vi "Gamepad PC.vi"() -> ()   [LabVIEW 2020]
uses:
  <vilib>/Utility/inputDevices.llb/closeJoystick.vi
panel:
  in  "stop":bool
  out "X Left":dbl(slide) scale=0.0..100.0
  out "nY Left":dbl(slide)
  out "Y Left":dbl(slide) scale=0.0..100.0
  out "nX Left":dbl(slide)
  out "X Right 2":dbl(slide) scale=0.0..100.0
  out "nY Right":dbl(slide)
  out "Z Left":dbl(slide)
  out "Z Right":dbl(slide) scale=0.0..100.0
  out "Y Right":dbl(slide) scale=0.0..100.0
  out "nX Right":dbl(slide)
  out "LB":bool
  out "RB":bool
  out "Back":bool
  out "Start":bool
  out "0":bool
  out "315":bool
  out "270":bool
  out "225":bool
  out "180":bool
  out "135":bool
  out "90":bool
  out "45":bool
  out "B":bool caption="Boolean"
  out "Y":bool caption="Boolean"
  out "A":bool caption="Boolean"
  out "X":bool caption="Boolean"
  out "R Stick":bool caption="Boolean"
  out "L Stick":bool caption="Boolean"
  out "error out":errorcluster
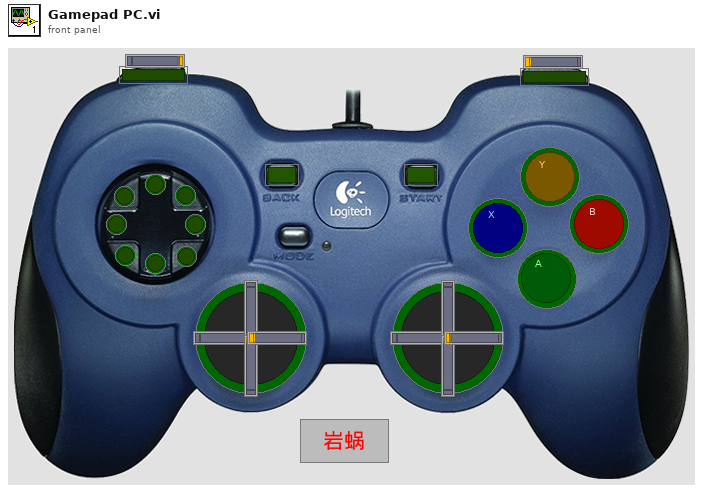
[diagram p1: front panel]
types:
  T1 = cluster{"axes total":u32, "buttons total":u32, "pov total":u32, "device name":string}[]
  T2 = typedef "Joystick controls.ctl" = cluster{"L Stick":bool, "R Stick":bool, "X":bool, "A":bool, "Y":bool, "B":bool, "45":bool, "90":bool, "135":bool, "180":bool, "225":bool, "270":bool, "315":bool, "0":bool, "Start":bool, "Back":bool, "RB":bool, "LB":bool, "X Right":i8, "Y Right":i8, "X Left":i8, "Y Left":i8, "Z Right":i8, "Pov":i16, "Z Left":i8, "Num":i16}
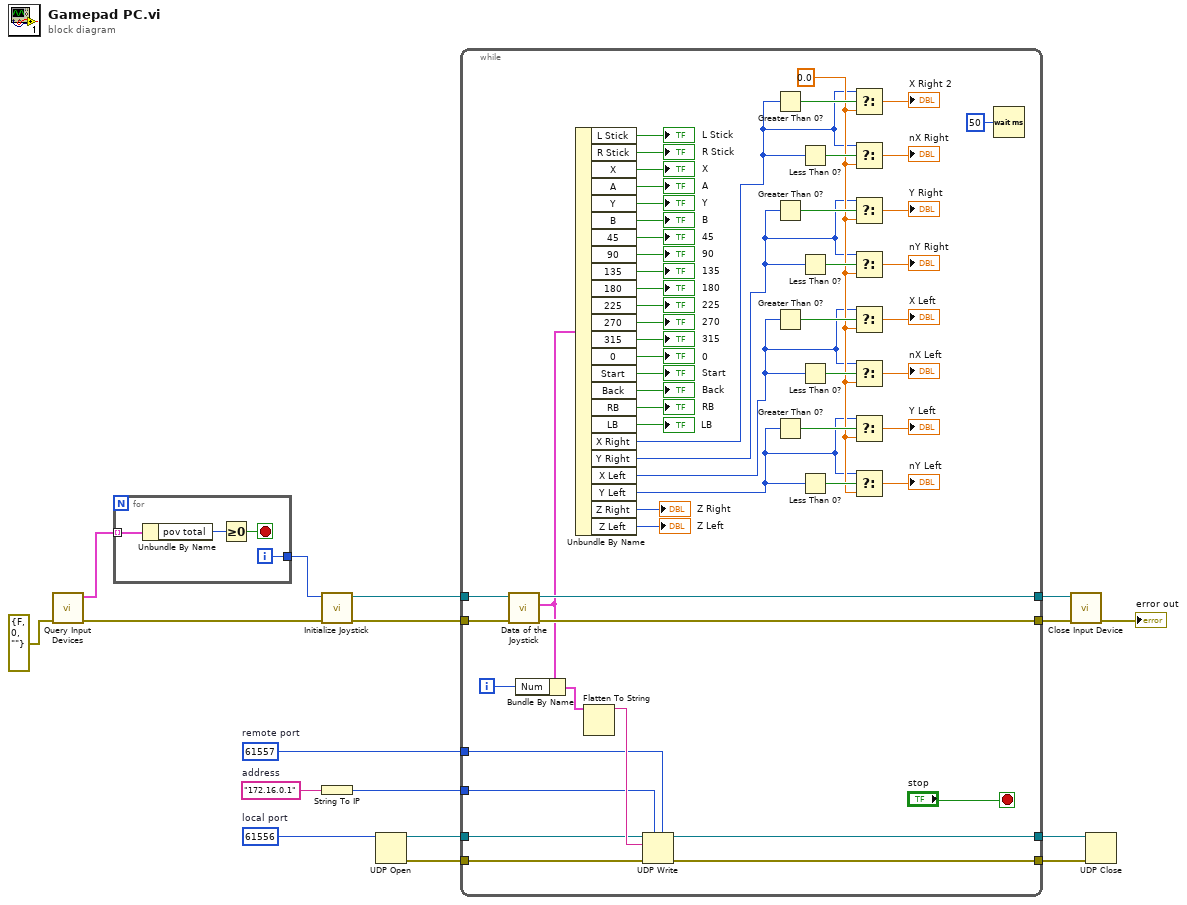
[diagram p0: block diagram]
diagram:
  w8 = "172.16.0.1"  # address
  w6 = u16 61557  # remote port
  w7 = u16 61556  # local port
  n1 = call <vilib>:"Query Input Devices.vi"("error in (no error)"=errorcluster {"status"=FALSE, "code"=0, "source"=""}) -> ("error out"=w9:errorcluster, "joystick info"=w11:T1)  [unwired: 7 in, 2 out]
  n2 = for {
    tunnel: w11 -> [w21] mode=indexing
    tunnel: [w18] -> w10
    i -> [w18]
    stop <- w20 stop-if-true
    n3 = Unbundle By Name(w21) -> ("pov total"=w19:u32)
    n4 = Greater Or Equal To 0?(x=w19) -> (x >= 0?=w20:bool)
  }
  n5 = call <vilib>:"Initialize Joystick.vi"("error in (no error)"=w9, "device index"=w10) -> ("error out"=w17:errorcluster, "device ID"=w14:refnum<k1>)  [unwired: 8 in]
  n6 = String To IP(1:w8) -> (0:w5:u32)
  n7 = UDP Open(11:w7) -> (port=w4:refnum<k16>, 0:w3:errorcluster)  [unwired: 4 in, 1 out]
  n8 = while {
    tunnel: w17 -> [w67]
    tunnel: [w66] -> w16
    tunnel: w14 -> [w68]
    tunnel: [w65] -> w13
    tunnel: w6 -> [w28]
    tunnel: w5 -> [w27]
    tunnel: w4 -> [w26]
    tunnel: w3 -> [w25]
    tunnel: [w23] -> w2
    tunnel: [w22] -> w1
    i -> [w30]
    stop <- "stop" stop-if-true
    w36 = 0.0 ("t")
    n9 = call "Data of the Joystick.vi"("error in (no error)"=w67, "device ID"=w68) -> ("error out"=w66:errorcluster, "Joystick"=w31:T2, "device ID out"=w65:refnum<k1>)  [unwired: 7 in]
    n10 = Bundle By Name(cluster=w31, "Num"=w30) -> (w24:T2)
    n11 = Unbundle By Name(w31) -> ("L Stick"=→"L Stick":bool, "R Stick"=→"R Stick":bool, "X"=→"X":bool, "A"=→"A":bool, "Y"=→"Y":bool, "B"=→"B":bool, "45"=→"45":bool, "90"=→"90":bool, "135"=→"135":bool, "180"=→"180":bool, "225"=→"225":bool, "270"=→"270":bool, "315"=→"315":bool, "0"=→"0":bool, "Start"=→"Start":bool, "Back"=→"Back":bool, "RB"=→"RB":bool, "LB"=→"LB":bool, "X Right"=w35:i8, "Y Right"=w34:i8, "X Left"=w33:i8, "Y Left"=w32:i8, "Z Right"=→"Z Right":i8, "Z Left"=→"Z Left":i8)
    n12 = Flatten To String(anything=w24) -> (data string=w29:string)  [unwired: 3 in, 2 out]
    n13 = UDP Write(address=w27, port or service name=w28, connection ID=w26, data in=w29, 8:w25) -> (error out=w23:errorcluster, 3:w22:refnum<k16>)  [unwired: 1 in]
    n14 = Greater Than 0?(x=w35) -> (x > 0?=w77:bool)
    n15 = Greater Than 0?(x=w34) -> (x > 0?=w75:bool)
    n16 = Greater Than 0?(x=w33) -> (x > 0?=w73:bool)
    n17 = Greater Than 0?(x=w32) -> (x > 0?=w71:bool)
    n18 = Less Than 0?(x=w35) -> (x < 0?=w76:bool)
    n19 = Less Than 0?(x=w34) -> (x < 0?=w74:bool)
    n20 = Less Than 0?(x=w33) -> (x < 0?=w72:bool)
    n21 = Less Than 0?(x=w32) -> (x < 0?=w70:bool)
    n22 = Select(t=w35, s=w77, f=w36) -> (s? t:f=→"X Right 2":dbl)
    n23 = Select(t=w35, s=w76, f=w36) -> (s? t:f=→"nX Right":dbl)
    n24 = Select(t=w34, s=w75, f=w36) -> (s? t:f=→"Y Right":dbl)
    n25 = Select(t=w34, s=w74, f=w36) -> (s? t:f=→"nY Right":dbl)
    n26 = Select(t=w33, s=w73, f=w36) -> (s? t:f=→"X Left":dbl)
    n27 = Select(t=w33, s=w72, f=w36) -> (s? t:f=→"nX Left":dbl)
    n28 = Select(t=w32, s=w71, f=w36) -> (s? t:f=→"Y Left":dbl)
    n29 = Select(t=w32, s=w70, f=w36) -> (s? t:f=→"nY Left":dbl)
    n30 = Wait (ms)(milliseconds to wait=u32 50) -> ()  [unwired: 1 out]
  }
  n31 = call-poly <vilib>:"Close Input Device.vi"("error in (no error)"=w16, "device ID"=w13) -> ("error out"=→"error out":errorcluster)  [unwired: 8 in]
  n32 = UDP Close(connection ID=w1, 8:w2) -> ()  [unwired: 2 out]
